vi "Write Configuration.vi"(8 "error in (no error)":errorcluster, 10 "Configuration.lvlibp:Configuration.lvclass":refnum<class "Configuration.lvclass">, 11 "Thermal Camera in":refnum<class "Thermal Camera.lvclass">) -> (0 "error out":errorcluster, 3 "Thermal Camera out":refnum<class "Thermal Camera.lvclass">)   [LabVIEW 2018, in "Thermal Camera.lvlib" / "Thermal Camera.lvclass"]
uses:
  Thermal Camera.lvclass
  PPLs/Configuration/Configuration.lvlibp/Configuration.lvclass
  Thermal Camera.lvclass/Thermal Camera.ctl
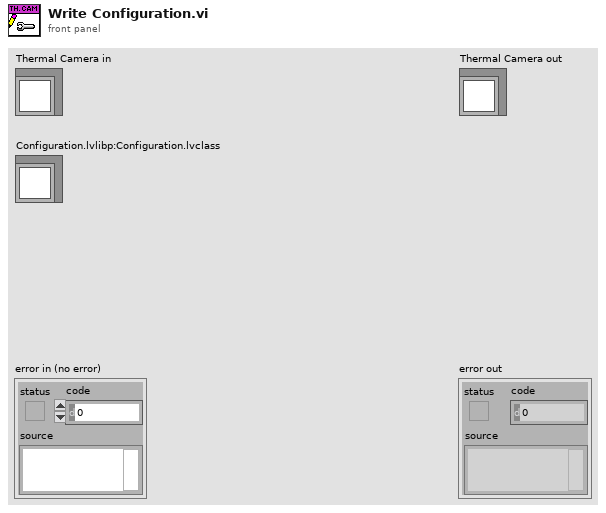
[diagram p1: front panel]
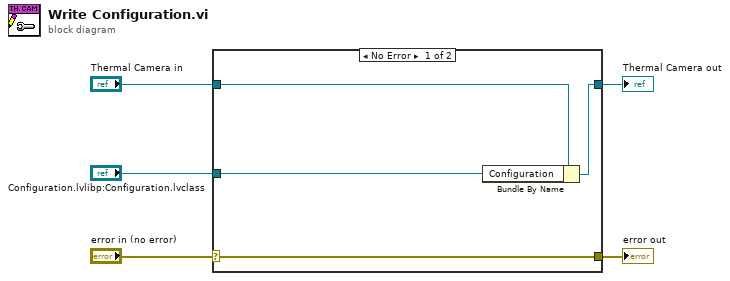
[diagram p0: block diagram]
diagram:
  n1 = case shown="No Error" "error in (no error)" {
    selector: "error in (no error)" -> [w9 w10]
    tunnel: [w9 w10] -> w4
    tunnel: [w7 w11] -> w2
    tunnel: "Thermal Camera in" -> [w8 w11]
    tunnel: "Configuration.lvlibp:Configuration.lvclass" -> [w6 _]
    frame No Error {
      n2 = Bundle By Name(cluster=w8, "Configuration"=w6) -> (w7:refnum<class "Thermal Camera.lvclass">)
    }
    frame Error {
    }
  }
  "error out" <- w4
  "Thermal Camera out" <- w2
